vi "Send Status.vi"(8 "error in (no error)":errorcluster, 10 "Status":string, 11 "QControl Creation in":refnum<class "QControl Creation.lvclass">) -> (0 "error out (dup)":errorcluster, 3 "QControl Creation (dup)":refnum<class "QControl Creation.lvclass">)   [LabVIEW 2023, in "QControl Creation.lvclass"]
doc: "<b> </b> <b> </b>\n©2016 Q Software Innovations, LLC (QSI)\nwritten by Quentin Alldredge\nproduced in LabVIEW 2015\n\nsupport@qsoftwareinnovations.com\nwww.qsoftwareinnovations.com\n\nAll rights reserved.\n\nRedistribution and use in source and binary forms, with or without modification, are permitted provided that the following conditions are met:\n\n * Redistributions of source code must retain the above copyright notice, this list of conditions and the following disclaimer.\n * Redistributions in binary form must reproduce the above copyright notice, this list of conditions and the following disclaimer in the documentation and/or other materials provided with the distribution.\n * Neither the name of Q Software Innovations, LLC. nor the names of its contributors may be used to endorse or promote products derived from this software without specific prior written permission.\n\nTHIS SOFTWARE IS PROVIDED BY THE COPYRIGHT HOLDERS AND CONTRIBUTORS \"AS IS\" AND ANY EXPRESS OR IMPLIED WARRANTIES, INCLUDING, BUT NOT LIMITED TO, THE IMPLIED WARRANTIES OF MERCHANTABILITY AND FITNESS FOR A PARTICULAR PURPOSE ARE DISCLAIMED. IN NO EVENT SHALL THE COPYRIGHT OWNER OR CONTRIBUTORS BE LIABLE FOR ANY DIRECT, INDIRECT, INCIDENTAL, SPECIAL, EXEMPLARY, OR CONSEQUENTIAL DAMAGES (INCLUDING, BUT NOT LIMITED TO, PROCUREMENT OF SUBSTITUTE GOODS OR SERVICES; LOSS OF USE, DATA, OR PROFITS; OR BUSINESS INTERRUPTION) HOWEVER CAUSED AND ON ANY THEORY OF LIABILITY, WHETHER IN CONTRACT, STRICT LIABILITY, OR TORT (INCLUDING NEGLIGENCE OR OTHERWISE) ARISING IN ANY WAY OUT OF THE USE OF THIS SOFTWARE, EVEN IF ADVISED OF THE POSSIBILITY OF SUCH DAMAGE."
uses:
  QControl Creation.lvclass
  QControl Creation.lvclass/QControl Creation.ctl
  New QControl Info/New QControl Info.lvclass/New QControl Info.ctl
  New QControl Info/Read StatusUpdate.vi
  New QControl Info/New QControl Info.lvclass
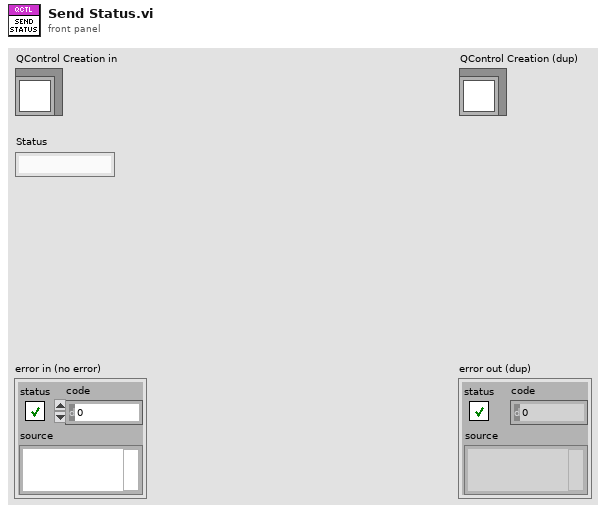
[diagram p1: front panel]
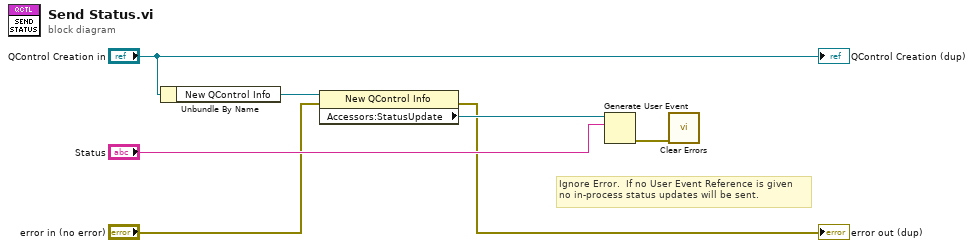
[diagram p0: block diagram]
diagram:
  # "Ignore Error.  If no User Event Reference is given\nno in-process status updates will be sent."
  n1 = Unbundle By Name("QControl Creation in") -> ("New QControl Info"=w6:refnum<data-value>)
  n2 = property class="New QControl Info"(reference=w6, error in="error in (no error)") -> (error out=→"error out (dup)":errorcluster, "Accessors:StatusUpdate"=w3:refnum<user-event>)  [unwired: 1 out]
  n3 = Generate User Event(user event=w3, event data cluster="Status") -> (error out=w4:errorcluster)  [unwired: 2 in, 1 out]
  n4 = call <vilib>:"Clear Errors.vi"("error in (no error)"=w4) -> ()  [unwired: 5 in, 2 out]
  "QControl Creation (dup)" <- "QControl Creation in"
